vi "From Sequence Ref.vi"(8 "error in (no error)":errorcluster, 11 "Sequence":refnum<k7>) -> (0 "error out":errorcluster, 3 "Sequence out":refnum<class "Sequence.lvclass">)   [LabVIEW 2020, in "TSnax.lvlib" / "Sequence.lvclass"]
uses:
  Sequence.lvclass
  Sequence.lvclass/Sequence.ctl
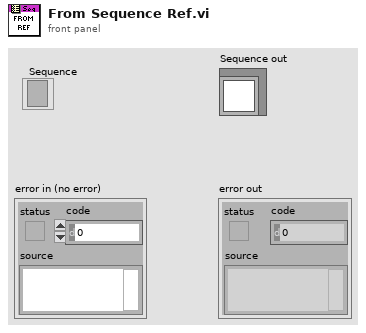
[diagram p1: front panel]
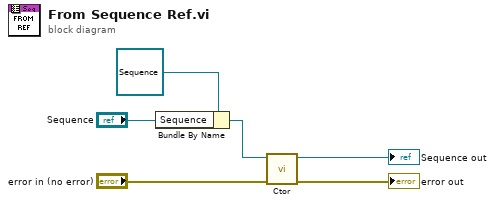
[diagram p0: block diagram]
diagram:
  n1 = Bundle By Name(cluster=refnum<class "Sequence.lvclass"> refnum ("Sequence in"), "Sequence"="Sequence") -> (w3:refnum<class "Sequence.lvclass">)
  n2 = call-dynamic "Ctor.vi"("error in (no error)"="error in (no error)", "Sequence in"=w3) -> ("error out"=→"error out":errorcluster, "Sequence out"=→"Sequence out":refnum<class "Sequence.lvclass">)  [unwired: 8 in]
